vi "PH_Timing.Action First Link Seq.vi"(0 "i ref in":refnum<vi>, 2 "Timing Mode":T1 {"T2" min=0 max=6000 step=2}, 5 "error IO":errorcluster) -> (14 "i ref out":refnum<vi>, 19 "error out":errorcluster)   [LabVIEW 2014, in "PH_Timing.lvlib"]
doc: "This is a certain process case of Timing."
uses:
  PH_Timing.lvlib
  PH_Timing.Timing Mode.ctl
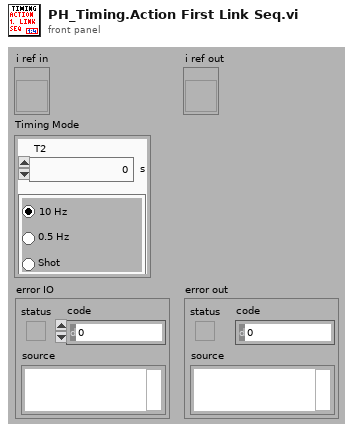
[diagram p1: front panel]
types:
  T1 = typedef "PH_Timing.lvlib/PH_Timing.Timing Mode.ctl" = cluster{"T2":i16, "Modeselector":enum32{"10 Hz", "0.5 Hz", "Shot"}}
  T2 = typedef "PH_Timing.lvlib/PH_Timing.i attribute.ctl" = cluster{"Sequencer":cluster{"linked?":bool, "Proc State":string, "Ref State":refnum<vi>}, "Gate Generator":cluster{"GD":cluster{"Device Status":T3, "linked?":bool}, "Settings":T4, "GUI Ref":refnum<vi>}, "Interlock Bypass":cluster{"Instancename":string, "Switch linked?":bool, "Device Status":T3, "Ref Status":refnum<vi>}, "Roughtuner":cluster{"Settings":T5, "GUI Ref":refnum<vi>, "GD":cluster{"Device Status":T3, "linked?":bool}}, "0,5Hz Gater":cluster{"Settings":T6, "GUI Ref":refnum<vi>, "GD":cluster{"Device Status":T3, "linked?":bool}}, "Slow Trigger":cluster{"Settings":T7, "GUI Ref":refnum<vi>, "Service ID Delay":i32, "Service ID Ext Trig":i32, "Wanted Settings":T7}, "Timing Mode":cluster{"Mode":T1, "GUI Ref":refnum<vi>, "Service ID T2":i32, "Service ID Mode":i32, "Wanted Mode":T1}, "ns Generator":cluster{"Settings":T8, "ns Generator Settings":refnum<vi>, "GD":cluster{"Device Status":T3, "linked?":bool}}, "Phase FEs":cluster{"Settings":T11, "GUI Ref":refnum<vi>, "Service ID Phase":i32, "Wanted Settings":T11}, "GD GUI Refs":refnum<vi>[], "Heads":T12[], "GUI Ref Delete":refnum<vi>}
  T3 = typedef "PH_StatusHandler.lvlib/PH_StatusHandler.Status.ctl" = i16
  T4 = typedef "PH_Timing.lvlib/PH_Timing.GateGen.ctl" = cluster{"Instance":string, "Channel Gate":i32, "Channel T2":i32, "Width Gate":dbl, "Width T2":dbl, "Delay Gate":dbl, "Delay T2":dbl, "Gate activ":bool, "T2 activ":bool, "System Mode":enum16{"Normal", "Single", "Burst", "Duty Cycle"}}
  T5 = typedef "PH_Timing.lvlib/PH_Timing.Roughtuner.ctl" = cluster{"Instance":string, "Phase PHELIX / UNILAC":cluster{"Channel":u16, "relative to":u16, "Delay [ms]":dbl}, "Pulse Length":cluster{"Channel":u16, "relative to":u16, "Delay [ms]":dbl}, "Trigger":cluster{"externally?":bool, "Rate [Hz]":dbl}}
  T6 = typedef "PH_Timing.lvlib/PH_Timing.0.5HzGater.ctl" = cluster{"Instance":string, "Channel ns FE Delay":i32, "Channel 0.5Hz":i32, "Width ns FE Delay":dbl, "Width 0.5Hz":dbl, "Delay ns FE Delay":dbl, "Delay 0.5Hz":dbl, "ns FE Delay active":bool, "0.5Hz activ":bool, "ns FE Delay inverted":bool, "0.5Hz inverted":bool}
  T7 = typedef "PH_Timing.lvlib/PH_Timing.Slow Trigger Settings.ctl" = cluster{"Delay":dbl, "externally triggered?":bool}
  T8 = typedef "PH_Timing.lvlib/PH_Timing.ns Generator.ctl" = cluster{"Instance":string, "Phase fs / ns FE":cluster{"Channel":T9, "Settings":T10}}
  T9 = typedef "Stanford Research DG645 - Driver.lvlib/Channel.ctl" = i32
  T10 = typedef "PH_SRDG645.lvlib/PH_SRDG645.Channel Settings.ctl" = cluster{"Delay [s]":dbl, "relative to":i32}
  T11 = typedef "PH_Timing.lvlib/PH_Timing.Phase FEs.ctl" = cluster{"Phase":dbl}
  T12 = typedef "PH_Timing.lvlib/PH_Timing.PU Data.ctl" = cluster{"linked?":bool, "Data":T13, "GD":cluster{"Device Status":T3, "linked?":bool}, "GUI Ref":refnum<vi>, "PU":T14}
  T13 = typedef "PH_Timing.lvlib/PH_Timing.PU Info.ctl" = cluster{"Act CH?":bool, "GD":string, "CH":i32, "Delay":dbl, "active":bool, "in Use?":bool}
  T14 = typedef "PH_PP_Common.lvlib/PH_PP_Common.PUs.ctl" = enum16{"no Info", "PA-19mm-1", "PA-19mm-2", "PA-45mm-PILC", "PA-45mm-MAIN", "MA-PU-1", "MA-PU-2", "MA-PU-3", "MA-PU-4", "MA-PU-5", "MA-PU-6", "MA-FR", "MA-PILC", "PA-45mm-DP"}
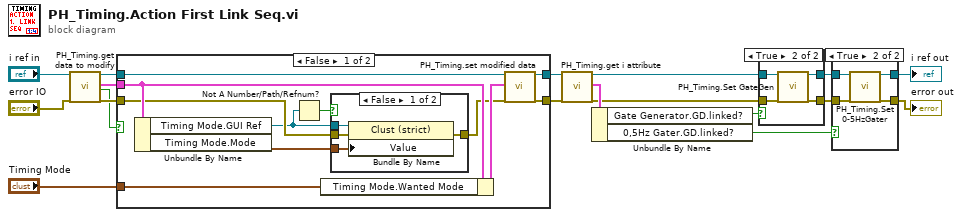
[diagram p0: block diagram]
diagram:
  n1 = call "PH_Timing.get data to modify.vi"("i ref in"="i ref in", "error in (no error)"="error IO") -> ("i ref out"=w18:refnum<vi>, "i attribute"=w16:T2, "timed out"=w15:bool, "error out"=w17:errorcluster)  [unwired: 14 in]
  n2 = case shown="False" w15 {
    tunnel: w18 -> [w29 w36]
    tunnel: [w28 w36] -> w9
    tunnel: w17 -> [w22 w35]
    tunnel: [w27 w35] -> w7
    tunnel: w16 -> [w24 _]
    tunnel: "Timing Mode" -> [w25 _]
    frame False {
      n3 = Unbundle By Name(w24) -> ("Timing Mode.GUI Ref"=w19:refnum<vi>, "Timing Mode.Mode"=w23:T1)
      n4 = Not A Number/Path/Refnum?(number/path/refnum=w19) -> (NaN/Path/Refnum?=w20:bool)
      n5 = Bundle By Name(cluster=w24, "Timing Mode.Wanted Mode"=w25) -> (w26:T2)
      n6 = case shown="False" w20 {
        tunnel: w19 -> [w33 _]
        tunnel: w23 -> [w32 _]
        tunnel: w22 -> [w31 w34]
        tunnel: [w30 w34] -> w21
        frame False {
          n7 = property class="Clust (strict)"(reference=w33, error in=w31, "Value"=w32) -> (error out=w30:errorcluster)  [unwired: 1 out]
        }
        frame True {
        }
      }
      n8 = call "PH_Timing.set modified data.vi"("i ref in"=w29, "i attribute"=w26, "error in (no error)"=w21) -> ("i ref out"=w28:refnum<vi>, "error out"=w27:errorcluster)  [unwired: 15 in]
    }
    frame True {
    }
  }
  n9 = call "PH_Timing.get i attribute.vi"("i ref in"=w9, "error in (no error)"=w7) -> ("i ref out"=w10:refnum<vi>, "i attribute"=w11:T2, "error out"=w8:errorcluster)  [unwired: 15 in]
  n10 = Unbundle By Name(w11) -> ("Gate Generator.GD.linked?"=w2:bool, "0,5Hz Gater.GD.linked?"=w1:bool)
  n11 = case shown="True" w2 {
    tunnel: [w38 w42] -> w5
    tunnel: [w37 w41] -> w3
    tunnel: w10 -> [w38 w40]
    tunnel: w8 -> [w37 w39]
    frame False {
    }
    frame True {
      n12 = call "PH_Timing.Set GateGen.vi"("i ref in"=w40, "error in (no error)"=w39) -> ("i ref out"=w42:refnum<vi>, "error out"=w41:errorcluster)  [unwired: 16 in]
    }
  }
  n13 = case shown="True" w1 {
    tunnel: [w44 w46] -> w6
    tunnel: w5 -> [w44 w48]
    tunnel: [w43 w45] -> w4
    tunnel: w3 -> [w43 w47]
    frame False {
    }
    frame True {
      n14 = call "PH_Timing.Set 0-5HzGater.vi"("i ref in"=w48, "error in (no error)"=w47) -> ("i ref out"=w46:refnum<vi>, "error out"=w45:errorcluster)  [unwired: 16 in]
    }
  }
  "i ref out" <- w6
  "error out" <- w4
